vi "Read All.vi"(6 "Per Read Size":u64=1024 max=30000, 8 "Error In":errorcluster, 10 "Max Read Size":u64=1024, 11 "Channel In":refnum<class "Channel.lvclass">=refnum) -> (0 "Error Out":errorcluster, 1 "Timed Out?":bool, 2 "Data":u8[](array[numeric]), 3 "Channel Out":refnum<class "Channel.lvclass">)   [LabVIEW 2021, in "Field_RnD_Services_LIBSSH2_Toolkit.lvlib" / "Channel.lvclass"]
doc: "Reads binary data from a SSH channel represented by this Channel object in chunks, or blocks, until the total read size is reached. This VI should be used if the <B>Total Read Size</B> is greater than 30KB because of a hard-coded per-read maximum of 30KB set in the libssh2 shared library."
uses:
  220524-VNA RP FLAT.llb/Channel.lvclass
  220524-VNA RP FLAT.llb/Session.lvclass
  220524-VNA RP FLAT.llb/SSH.lvclass
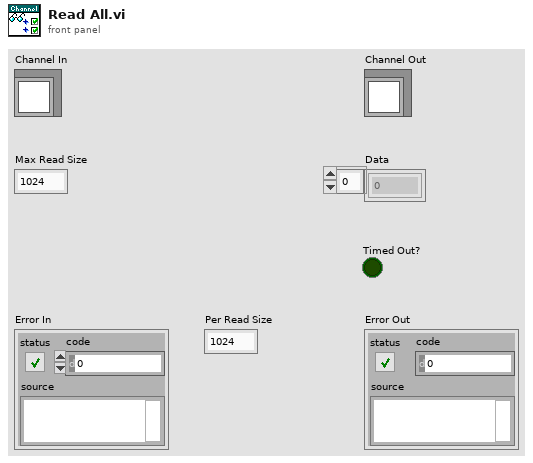
[diagram p1: front panel]
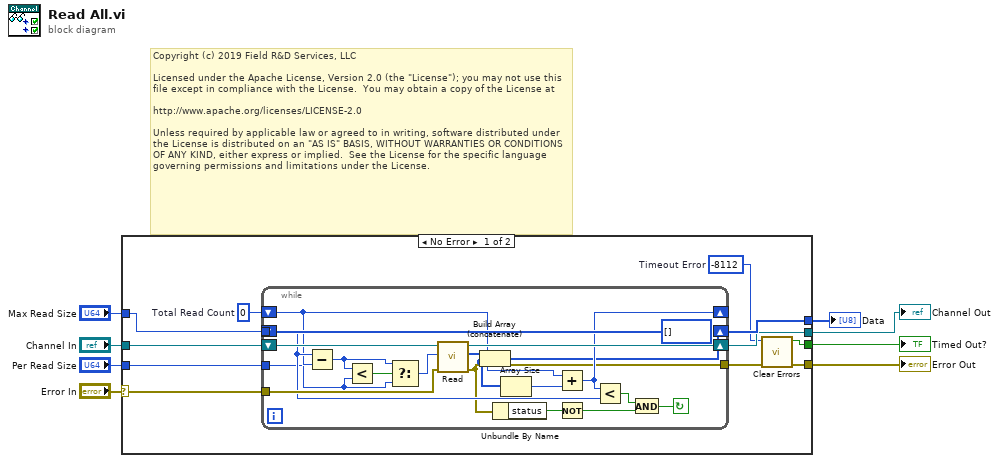
[diagram p0: block diagram]
diagram:
  # "Copyright (c) 2019 Field R&D Services, LLC\n\nLicensed under the Apache License, Version 2.0 (the \"License\"); you may not use this file except in compliance with the License.  You may obtain a copy of the License at\n\nhttp://www.apache.org/licenses/LICENSE-2.0\n\nUnless required by applicable law or agreed to in writing, software distributed under the License is distributed on an \"AS IS\" BASIS, WITHOUT WARRANTIES OR CONDITIONS OF ANY KIND, either express or implied.  See the License for the specific language governing permissions and limitations under the License."
  n1 = case shown="No Error" "Error In" {
    selector: "Error In" -> [w14 w40]
    tunnel: "Max Read Size" -> [w19 _]
    tunnel: "Per Read Size" -> [w18 _]
    tunnel: "Channel In" -> [w17 w41]
    tunnel: [w16 _] -> w5
    tunnel: [w15 w41] -> w4
    tunnel: [w12 w40] -> w3
    tunnel: [w10 _] -> w1
    frame No Error {
      w11 = -8112  # Timeout Error
      w20 = u64 0  # Total Read Count
      n2 = while {
        shift-right: [w37] -> w15
        shift-left: w17 -> [w39]
        shift-right: [w34] -> _
        shift-left: w20 -> [w32]
        tunnel: w19 -> [w33]
        tunnel: w18 -> [w28]
        tunnel: w14 -> [w38]
        tunnel: [w27] -> w13
        shift-right: [w21] -> w16
        shift-left: u8[] [] ("Data") -> [w22]
        stop <- w23 continue-if-true
        n3 = Subtract(x=w33, y=w32) -> (x-y=w30:u64)
        n4 = Less?(x=w30, y=w28) -> (x < y?=w31:bool)
        n5 = Select(t=w30, s=w31, f=w28) -> (s? t:f=w29:u64)
        n6 = call "Read.vi"("Error In"=w38, "Max Data Length"=w29, "Channel In"=w39) -> ("Error Out"=w27:errorcluster, "Data"=w36:u8[], "Channel Out"=w37:refnum<class "Channel.lvclass">)  [unwired: 6 in]
        n7 = Build Array (concatenate)(w22, w36) -> (w21:u8[])
        n8 = Unbundle By Name(w27) -> ("status"=w26:bool)
        n9 = Array Size(array=w36) -> (size(s)=w35:i32)
        n10 = Add(x=w32, y=w35) -> (x+y=w34:u64)
        n11 = Not(x=w26) -> (.not. x?=w24:bool)
        n12 = Less?(x=w34, y=w33) -> (x < y?=w25:bool)
        n13 = And(x=w25, y=w24) -> (x .and. y?=w23:bool)
      }
      n14 = call <vilib>:"Clear Errors.vi"("error in (no error)"=w13, "specific error code to clear (0: all)"=w11) -> ("error out"=w12:errorcluster, "specific error cleared?"=w10:bool)  [unwired: 4 in]
    }
    frame Error {
    }
  }
  "Data" <- w5
  "Channel Out" <- w4
  "Error Out" <- w3
  "Timed Out?" <- w1
